vi "Launch Test Actors.vi"   [LabVIEW 2015]
uses:
  Load App.vi
  Test Actors.lvclass
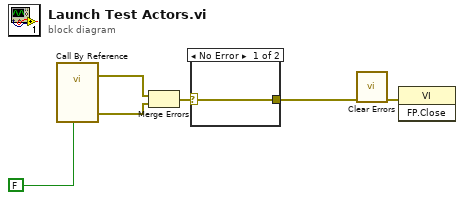
[diagram p0: block diagram]
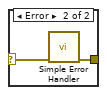
[diagram p2: hidden frame]
diagram:
  n1 = call-by-ref "?"("Open Actor Core front panel? (F)"=FALSE) -> (error out=w4:errorcluster, "Error Out"=w3:errorcluster)  [unwired: 12 in, 1 out]
  n2 = Merge Errors(w4, w3) -> (w5:errorcluster)
  n3 = case shown="No Error" w5 {
    selector: w5 -> [w7 w9]
    tunnel: [w7 w8] -> w1
    frame No Error {
    }
    frame Error {
      n4 = call <vilib>:"Simple Error Handler.vi"("error in (no error)"=w9) -> ("error out"=w8:errorcluster)  [unwired: 4 in, 4 out]
    }
  }
  n5 = call <vilib>:"Clear Errors.vi"("error in (no error)"=w1) -> ("error out"=w6:errorcluster)  [unwired: 5 in, 1 out]
  n6 = invoke class="VI" method="FP.Close"(error in=w6) -> ()  [unwired: 2 in, 3 out]
